vi "test Log Span Size.vi"(8 "error in":errorcluster, 11 "TestCase in":refnum<class "Embedded Data Logger Windows System Tests.lvclass">) -> (0 "error out":errorcluster, 3 "TestCase out":refnum<class "Embedded Data Logger Windows System Tests.lvclass">)   [LabVIEW 2027, in "Embedded Data Logger Windows System Tests.lvclass"]
uses:
  Embedded Data Logger Windows System Tests.lvclass
  C:/Program Files/National Instruments/LabVIEW 2027/vi.lib/addons/_JKI Toolkits/VI Tester/TestCase.llb/TestCase.lvclass
  <vilib>/addons/_JKI Toolkits/VI Tester/TestCase.llb/TestCase.lvclass
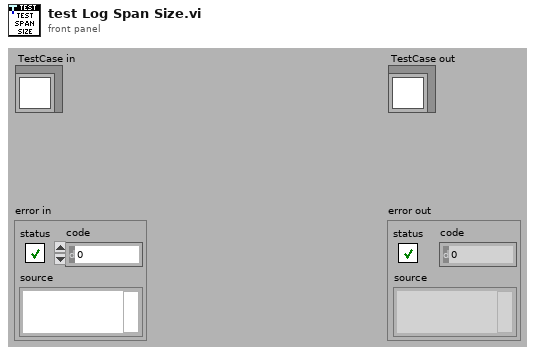
[diagram p1: front panel]
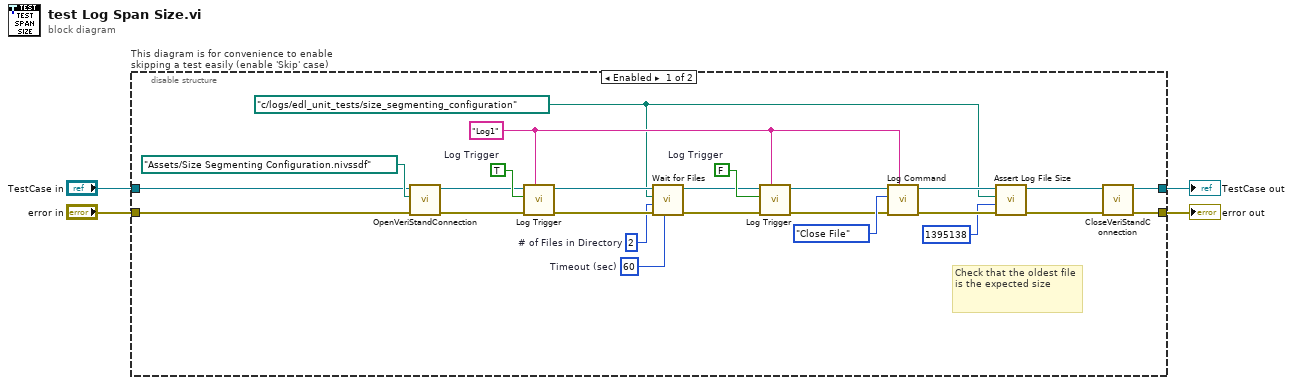
[diagram p0: block diagram]
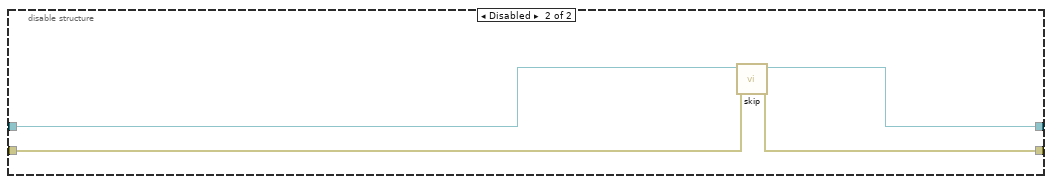
[diagram p2: hidden frame]
diagram:
  n1 = disable-structure "This diagram is for convenience to enable skipping a test easily (enable 'Skip' case)" shown="Enabled" {
    disable-tunnel: "TestCase in" -> [w17 w33]
    disable-tunnel: [w14 w31] -> w1
    disable-tunnel: [w13 w32] -> w3
    disable-tunnel: "error in" -> [w16 w30]
    frame Enabled {
      w5 = u32 60  # Timeout (sec)
      w6 = 2  # # of Files in Directory
      w7 = path "c:/logs/edl_unit_tests/size_segmenting_configuration" ("file path")
      w24 = "Log1" ("Embedded Data Logger File Name")
      w29 = FALSE  # Log Trigger
      w28 = TRUE  # Log Trigger
      # "Check that the oldest file is the expected size"
      n2 = call-dynamic "OpenVeriStandConnection.vi"("error in (no error)"=w16, "System Definition File"=path "Assets/Size Segmenting Configuration.nivssdf", "VeriStand Test Case in"=w17) -> ("error out"=w19:errorcluster, "VeriStand Test Case out"=w18:refnum<class "Embedded Data Logger Windows System Tests.lvclass">)  [unwired: 6 in, 1 out]
      n3 = call "Log Trigger.vi"("Embedded Data Logger File Name"=w24, "error in"=w19, "Log Trigger"=w28, "Embedded Data Logger System Tests in"=w18) -> ("error out"=w11:errorcluster, "Embedded Data Logger System Tests out"=w10:refnum<class "Embedded Data Logger Windows System Tests.lvclass">)  [unwired: 6 in]
      n4 = call "Wait for Files.vi"("Timeout (sec)"=w5, "Error In"=w11, "# of Files in Directory"=w6, "Log Directory"=w7, "TestCase in"=w10) -> ("Error Out"=w8:errorcluster, "TestCase out"=w9:refnum<class "Embedded Data Logger Windows System Tests.lvclass">)  [unwired: 5 in]
      n5 = call "Log Trigger.vi"("Embedded Data Logger File Name"=w24, "error in"=w8, "Log Trigger"=w29, "Embedded Data Logger System Tests in"=w9) -> ("error out"=w26:errorcluster, "Embedded Data Logger System Tests out"=w25:refnum<class "Embedded Data Logger Windows System Tests.lvclass">)  [unwired: 6 in]
      n6 = call "Log Command.vi"("Embedded Data Logger File Name"=w24, "error in"=w26, "Log Command"=enum16{"Idle", "Open File", "Close File"}."Close File", "Embedded Data Logger System Tests in"=w25) -> ("error out"=w22:errorcluster, "Embedded Data Logger System Tests out"=w23:refnum<class "Embedded Data Logger Windows System Tests.lvclass">)  [unwired: 6 in]
      n7 = call "Assert Log File Size.vi"("error in"=w22, "Expected size of file in bytes"=i64 1395138, "file path"=w7, "Embedded Data Logger System Tests in"=w23) -> ("error out"=w12:errorcluster, "Embedded Data Logger System Tests out"=w15:refnum<class "Embedded Data Logger Windows System Tests.lvclass">)  [unwired: 6 in]
      n8 = call-dynamic "CloseVeriStandConnection.vi"("error in (no error)"=w12, "VeriStand Test Case in"=w15) -> ("error out"=w13:errorcluster, "VeriStand Test Case out"=w14:refnum<class "Embedded Data Logger Windows System Tests.lvclass">)  [unwired: 8 in]
    }
    frame Disabled {
      # "skip test result while test is under development"
      n9 = call <vilib>:"skip.vi"("error in (no error)"=w30, "TestCase in"=w33) -> ("error out"=w32:errorcluster, "TestCase out"=w31:refnum<class "Embedded Data Logger Windows System Tests.lvclass">)  [unwired: 8 in]
    }
  }
  "error out" <- w3
  "TestCase out" <- w1
